vi "RTS Door Ops 2nd.vi"(4 "Relay Number":u8=1 min=1 max=3 step=1, 5 "Delay":bool, 6 "Door Open Delay(sec)":dbl, 7 "Door Open Sequence:":T1, 8 "error in (no error)":errorcluster, 10 "Current Status":string[](array[string]), 11 "Station 1-8 Data in in":T2 {"Station Slide"."Chamber 1-1"."Start Time" format="%<%X\n%x>T"; "Station Slide"."Chamber 1-1"."End Time" format="%<%X\n%x>T"; "Station Slide"."Time Count (s)" format="%.2f"; "Station Cab"."Chamber 1-1"."Start Time" format="%<%X\n%x>T"; "Station Cab"."Chamber 1-1"."End Time" format="%<%X\n%x>T"; "Station Cab"."Time Count (s)" format="%.2f"; "Station Freezer"."Chamber 1-1"."Start Time" format="%<%X\n%x>T"; "Station Freezer"."Chamber 1-1"."End Time" format="%<%X\n%x>T"; "Station Freezer"."Time Count (s)" format="%.2f"}) -> (0 "error out":errorcluster, 1 "Elapsed Time (sec)":dbl, 2 "Run Door Ops":bool, 3 "Station 1-8 Data out":T2 {"Station Slide"."Chamber 1-1"."Start Time" format="%<%X\n%x>T"; "Station Slide"."Chamber 1-1"."End Time" format="%<%X\n%x>T"; "Station Slide"."Time Count (s)" format="%.2f"; "Station Cab"."Chamber 1-1"."Start Time" format="%<%X\n%x>T"; "Station Cab"."Chamber 1-1"."End Time" format="%<%X\n%x>T"; "Station Cab"."Time Count (s)" format="%.2f"; "Station Freezer"."Chamber 1-1"."Start Time" format="%<%X\n%x>T"; "Station Freezer"."Chamber 1-1"."End Time" format="%<%X\n%x>T"; "Station Freezer"."Time Count (s)" format="%.2f"})   [LabVIEW 2016]
uses:
  Type Definitions/RTS Station Relay Ops.ctl
  Type Definitions/RTS Door Opener Indicator.ctl
  Type Definitions/RTS Door Ops Client.ctl
  Type Definitions/RTS Door Opening Schedule.ctl
  Type Definitions/RTS Door Ops Sequence.ctl
panel:
  out "Time has Elapsed":bool
  # "Chamber Conditions:"
  # "Chamber Conditions:"
  # "Chamber Conditions:"
  # "Chamber Conditions:"
  # "Chamber Conditions:"
  # "Chamber Conditions:"
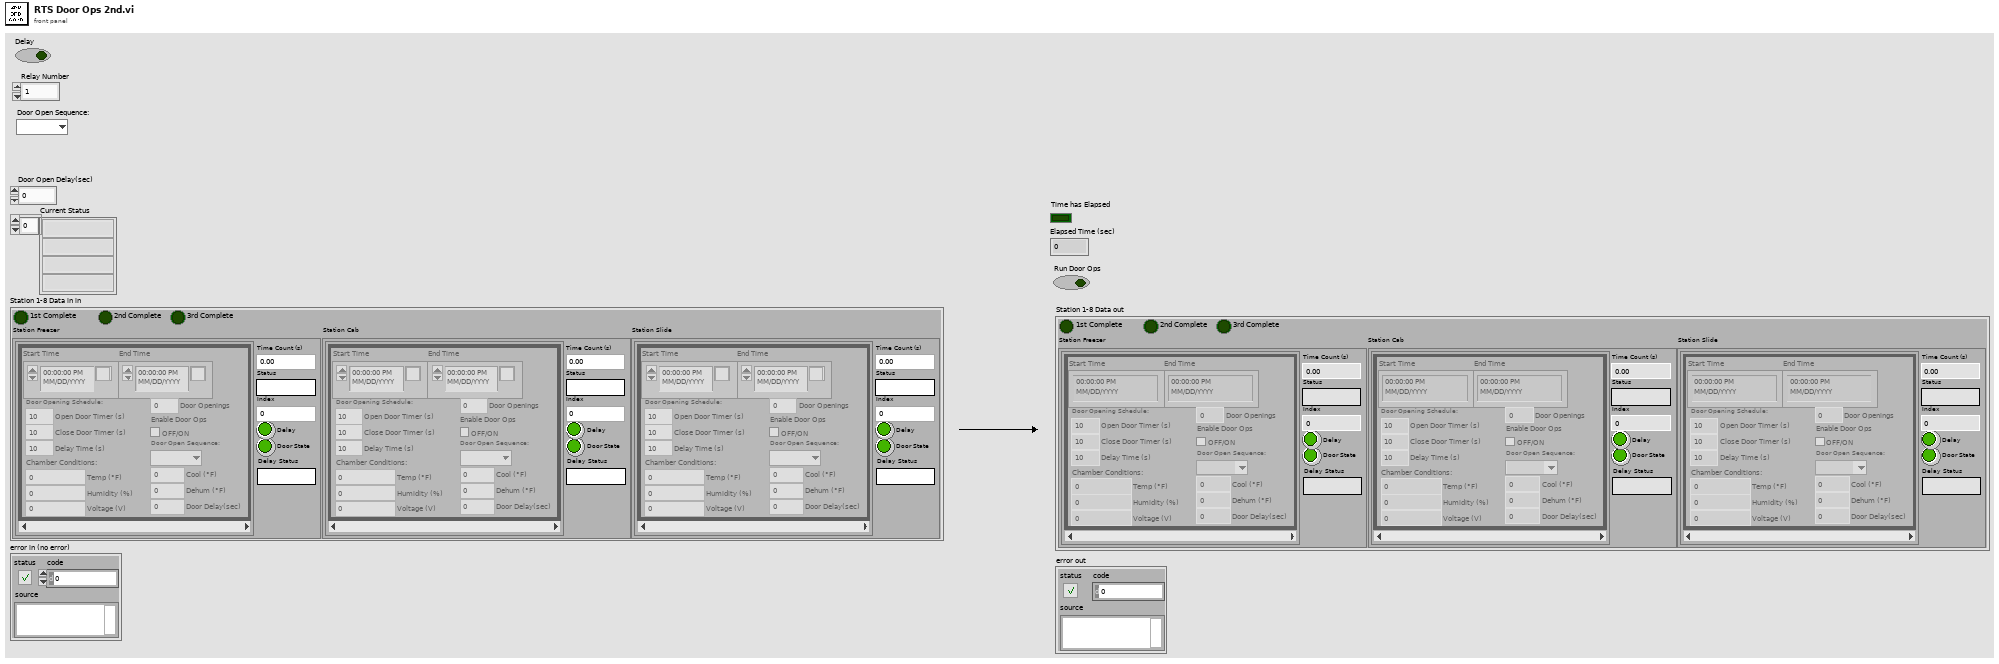
[diagram p1: front panel]
types:
  T1 = typedef "RTS Door Ops Sequence.ctl" = enum16{"", "1st", "2nd", "3rd"}
  T2 = typedef "RTS Station Relay Ops.ctl" = cluster{"Station Freezer":T3, "Station Cab":T3, "Station Slide":T3, "1st Complete":bool, "2nd Complete":bool, "3rd Complete":bool}
  T3 = typedef "RTS Door Opener Indicator.ctl" = cluster{"Time Count (s)":dbl, "Status":string, "Door State":bool, "Delay":bool, "Chamber 1-1":T4[], "Index":i32, "Delay Status":string}
  T4 = typedef "RTS Door Ops Client.ctl" = cluster{"End Time":timestamp, "Start Time":timestamp, "Door Opening Schedule:":T5, "Enable Door Ops":bool, "Door Openings":u32, "Temp (°F)":dbl, "Humidity (%)":dbl, "Voltage (V)":dbl, "Door Open Sequence:":T1, "Door Delay(sec)":dbl, "Dehum (°F)":dbl, "Cool (°F)":dbl}
  T5 = typedef "RTS Door Opening Schedule.ctl" = cluster{"Open Door Timer (s)":dbl, "Delay Time (s)":dbl, "Close Door Timer (s)":dbl}
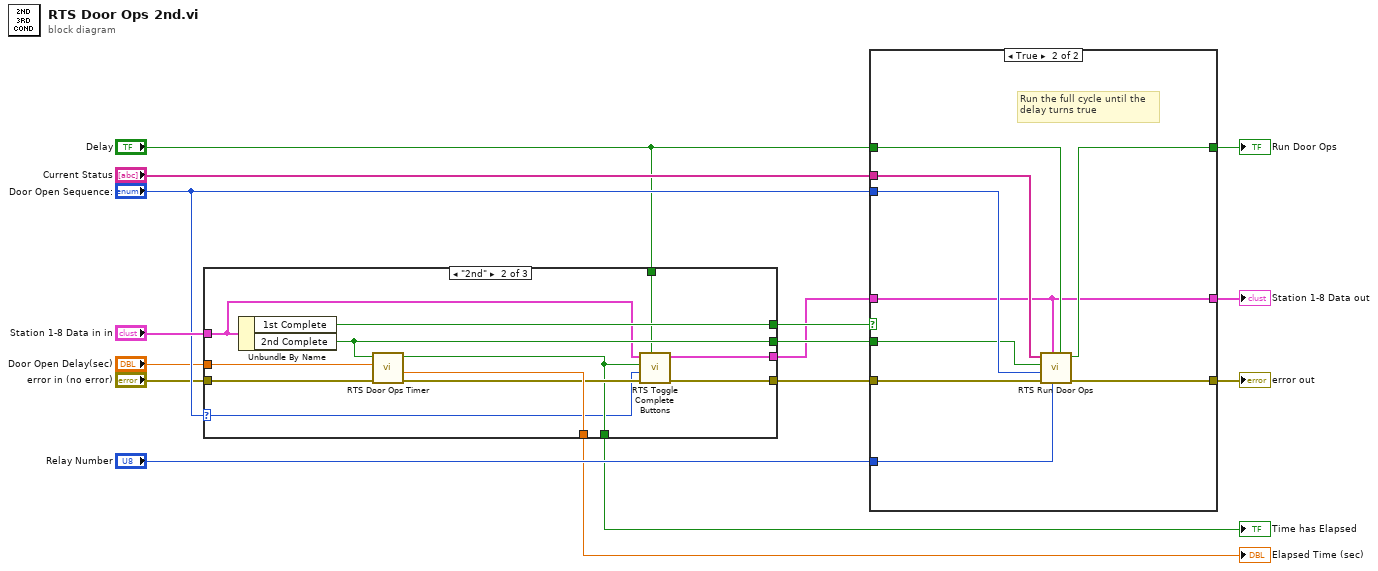
[diagram p0: block diagram]
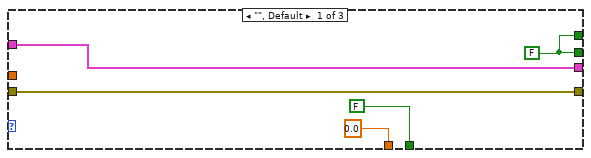
[diagram p2: hidden frame]
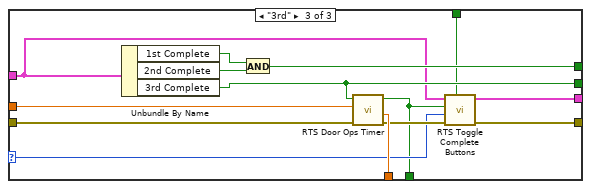
[diagram p3: hidden frame]
diagram:
  n1 = case shown="\"2nd\"" "Door Open Sequence:" {
    selector: "Door Open Sequence:" -> [_ w23 w36]
    tunnel: "Station 1-8 Data in in" -> [w18 w25 w37]
    tunnel: [w19 w33 w45] -> w11
    tunnel: [w19 w31 w41] -> w8
    tunnel: [0.0 ("Elapsed Time (sec)") w32 w42] -> w7
    tunnel: "error in (no error)" -> [w21 w30 w44]
    tunnel: [w21 w27 w39] -> w5
    tunnel: "Door Open Delay(sec)" -> [_ w29 w43]
    tunnel: "Delay" -> [_ w22 w38]
    tunnel: [FALSE ("Time has Elapsed") w24 w35] -> w2
    tunnel: [w18 w26 w34] -> w1
    frame "", Default {
      w19 = FALSE ("1st Complete")
    }
    frame "2nd" {
      n2 = Unbundle By Name(w25) -> ("1st Complete"=w33:bool, "2nd Complete"=w31:bool)
      n3 = call "RTS Door Ops Timer.vi"("Error In"=w30, "Door Open Delay(sec)"=w29, "Routine Complete"=w31) -> ("Error Out"=w28:errorcluster, "Elapsed Time (sec)"=w32:dbl, "Time has Elapsed"=w24:bool)  [unwired: 6 in]
      n4 = call "RTS Toggle Complete Buttons.vi"("Delay"=w22, "Error In"=w28, "Door Open Sequence:"=w23, "Times Up?"=w24, "Station 1-8 Data in in"=w25) -> ("Error Out"=w27:errorcluster, "Station 1-8 Data in out"=w26:T2)  [unwired: 5 in]
    }
    frame "3rd" {
      n5 = Unbundle By Name(w37) -> ("1st Complete"=w47:bool, "2nd Complete"=w46:bool, "3rd Complete"=w41:bool)
      n6 = And(x=w47, y=w46) -> (x .and. y?=w45:bool)
      n7 = call "RTS Door Ops Timer.vi"("Error In"=w44, "Door Open Delay(sec)"=w43, "Routine Complete"=w41) -> ("Error Out"=w40:errorcluster, "Elapsed Time (sec)"=w42:dbl, "Time has Elapsed"=w35:bool)  [unwired: 6 in]
      n8 = call "RTS Toggle Complete Buttons.vi"("Delay"=w38, "Error In"=w40, "Door Open Sequence:"=w36, "Times Up?"=w35, "Station 1-8 Data in in"=w37) -> ("Error Out"=w39:errorcluster, "Station 1-8 Data in out"=w34:T2)  [unwired: 5 in]
    }
  }
  "Elapsed Time (sec)" <- w7
  "Time has Elapsed" <- w2
  n9 = case shown="True" w11 {
    tunnel: w5 -> [w49 w53]
    tunnel: [w49 w51] -> w12
    tunnel: [w48 w59] -> w13
    tunnel: w1 -> [w50 w52]
    tunnel: [w50 w52] -> w15
    tunnel: w8 -> [_ w54]
    tunnel: "Current Status" -> [_ w56]
    tunnel: "Door Open Sequence:" -> [_ w58]
    tunnel: "Relay Number" -> [_ w55]
    tunnel: "Delay" -> [w48 w57]
    frame False {
      # "Wait for the 1st to complete"
    }
    frame True {
      # "Run the full cycle until the\ndelay turns true"
      n10 = call "RTS Run Door Ops.vi"("Delay"=w57, "Relay Number"=w55, "Station 1-8 Data in"=w52, "Error In"=w53, "Door Open Sequence:"=w58, "Complete?"=w54, "Current Status"=w56) -> ("Error Out"=w51:errorcluster, "Run Door Ops"=w59:bool)  [unwired: 2 in, 1 out]
    }
  }
  "Station 1-8 Data out" <- w15
  "Run Door Ops" <- w13
  "error out" <- w12
